vi "get Position.vi"(11 "Element in":refnum<class "Element.lvclass">) -> (3 "Position":refnum<class "Vector 2D.lvclass">)   [LabVIEW 2021, in "Element.lvclass"]
uses:
  Element.lvclass
  Re-use Libraries/Vector 2D/Vector 2D.lvclass
  Element.lvclass/Element.ctl
  Motion/Motion.lvclass
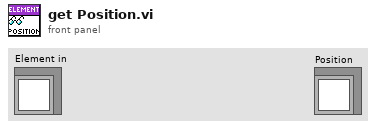
[diagram p1: front panel]
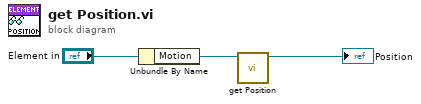
[diagram p0: block diagram]
diagram:
  n1 = Unbundle By Name("Element in") -> ("Motion"=w2:refnum<class "Motion.lvclass">)
  n2 = call "get Position.vi"("Motion in"=w2) -> ("Displacement"=→"Position":refnum<class "Vector 2D.lvclass">)  [unwired: 10 in]
